vi "Wait.Gui.vi"() -> ()   [LabVIEW 2016]
uses:
  Wait.Gui.Action.ctl
  Global/ApplicationGlobal.vi
panel:
  in  "Open?":bool
  out "message":string
  out "_loop":i32(ring)=4
  out "status":string
  out "Slide":i32(slide) scale=-1.1..-1.0
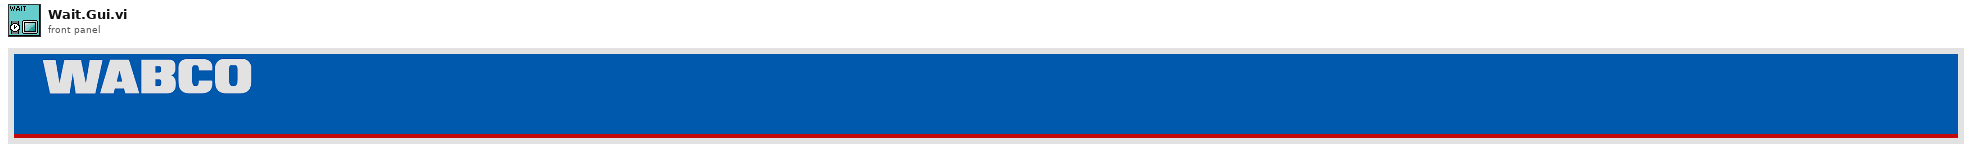
[diagram p1: front panel]
types:
  T1 = enum32{"Invalid", "Standard", "Closed", "Hidden", "Minimized", "Maximized"}
  T2 = enum32{"Invalid", "Default", "Floating", "Floating/Auto-Hide", "Modal"}
  T3 = cluster{"Msg":string, "Status":string, "ProgBarSize":i32, "Delay at open":u32}
  T4 = typedef "Wait.Gui.Action.ctl" = enum32{"idle", "constructor", "destructor", "--- WaitGui ---", "open FP", "close FP", "update msg", "update progbar"}
  T5 = typedef "LVPositionTypeDef.ctl" = cluster{"Left":i32, "Top":i32}
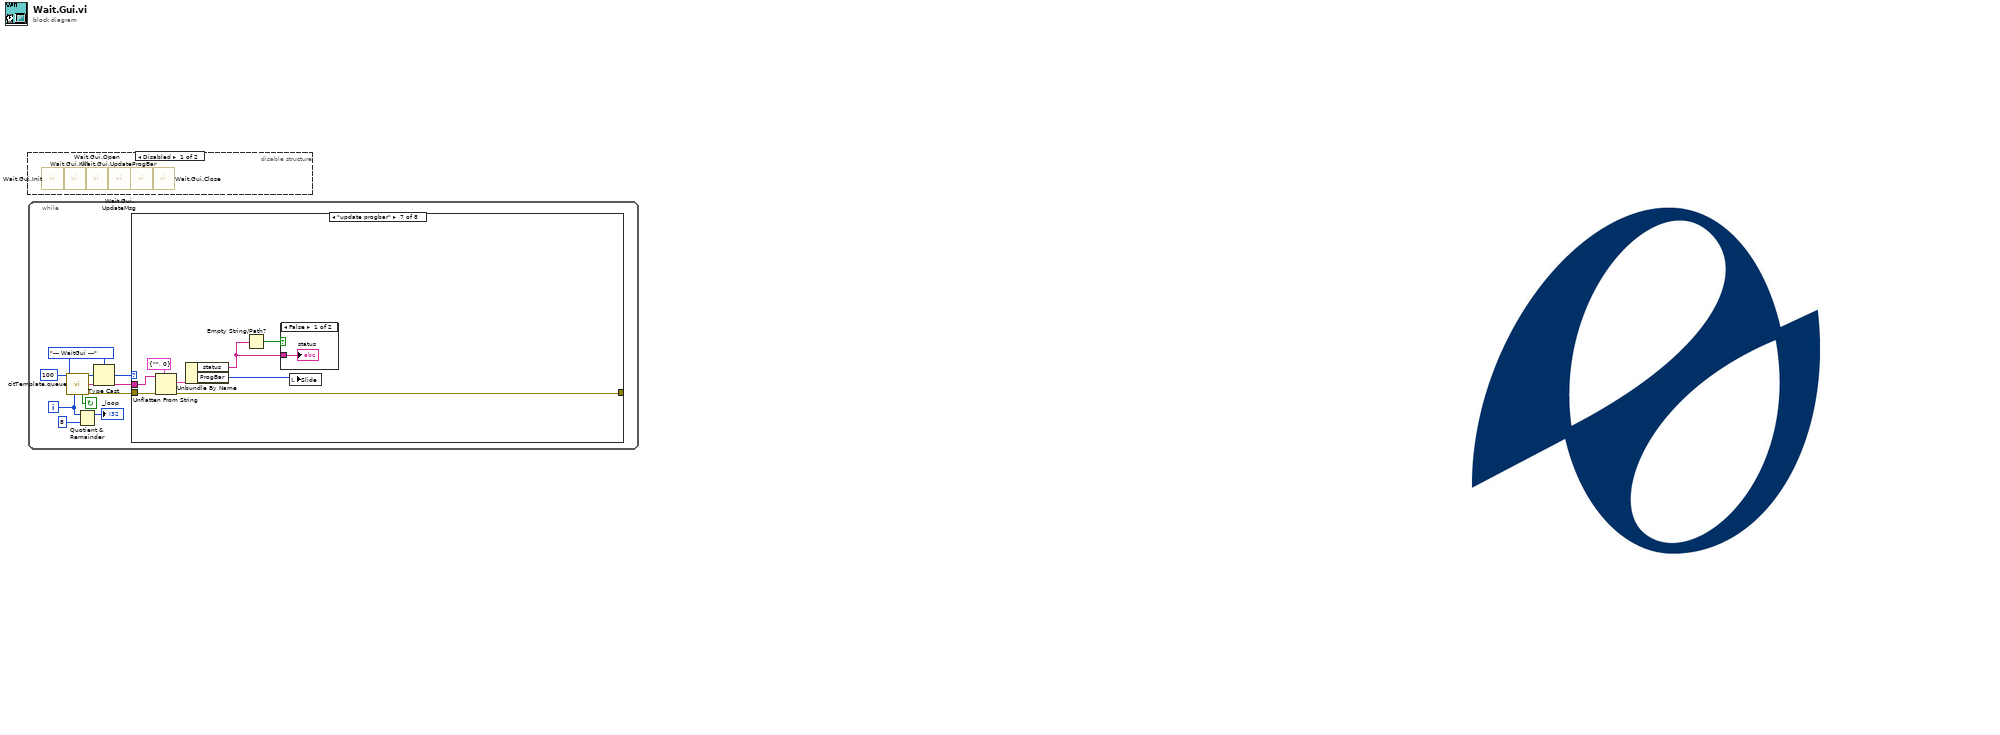
[diagram p0: block diagram]
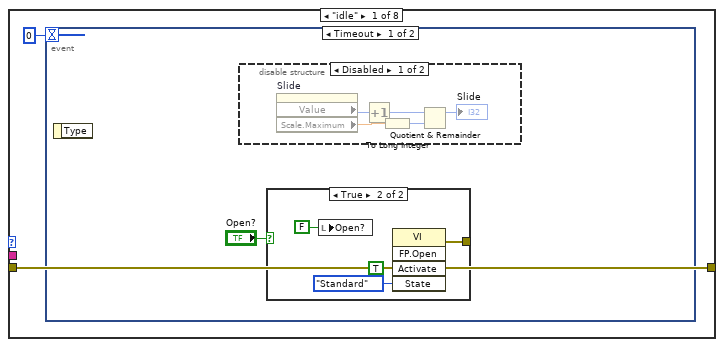
[diagram p3: hidden frame]
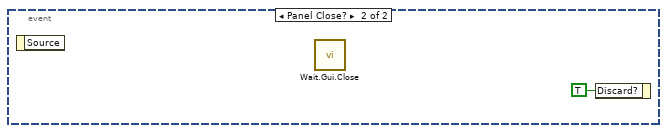
[diagram p6: hidden frame]
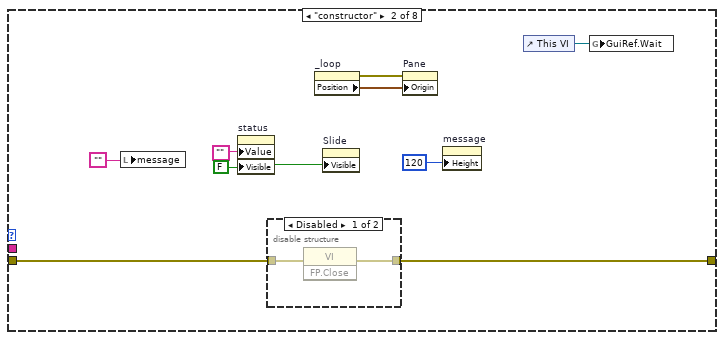
[diagram p7: hidden frame]
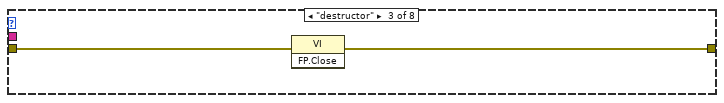
[diagram p9: hidden frame]
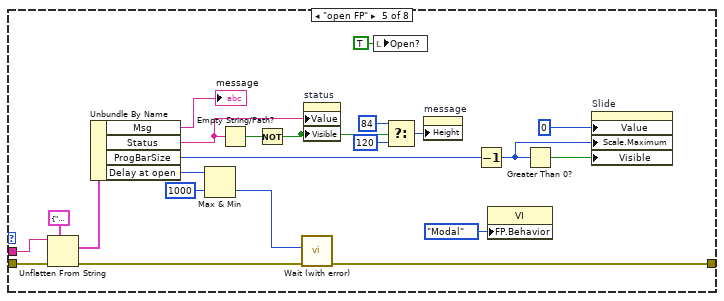
[diagram p11: hidden frame]
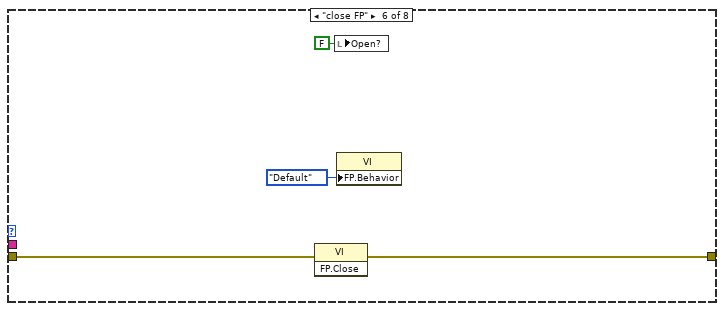
[diagram p12: hidden frame]
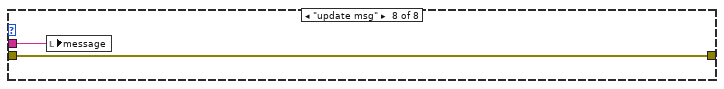
[diagram p14: hidden frame]
diagram:
  n1 = disable-structure shown="Disabled" {
    frame Disabled {
      n2 = call "Wait.Gui.Init.vi"() -> ()  [unwired: 11 in, 1 out]
      n3 = call "Wait.Gui.Kill.vi"() -> ()  [unwired: 11 in, 1 out]
      n4 = call "Wait.Gui.Open.vi"() -> ()  [unwired: 11 in, 1 out]
      n5 = call "Wait.Gui.UpdateMsg.vi"() -> ()  [unwired: 11 in, 1 out]
      n6 = call "Wait.Gui.UpdateProgBar.vi"() -> ()  [unwired: 11 in, 1 out]
      n7 = call "Wait.Gui.Close.vi"() -> ()  [unwired: 11 in, 1 out]
    }
    frame Enabled {
    }
  }
  n8 = while {
    i -> [w2]
    stop <- w4 continue-if-true
    w5 = Wait.Gui.Action."--- WaitGui ---" ("Action")
    n9 = call "citTemplate.queue.vi"("ms timeout (250 ms)"=100, "event enum"=w5, "iteration (-1)"=w2) -> ("event out"=w9:u32, "(flatten) data out"=w6:string, "continue"=w4:bool, "error out"=w7:errorcluster)  [unwired: 2 in, 7 out]
    n10 = Quotient & Remainder(x=w2, y=8) -> (x-y*floor(x/y)=→"_loop":i32)  [unwired: 1 out]
    n11 = Type Cast(type=w5, x=w9) -> (*(type *) &x=w8:T4)
    n12 = case shown="\"update progbar\"" w8 {
      tunnel: w7 -> [w11 w30 w37 w38 w60 w64 w72 w74]
      tunnel: w6 -> [_ _ _ _ w58 _ w71 w75]
      tunnel: [w11 w29 w36 w38 w42 w63 w70 w74] -> _
      frame "idle" {
        n13 = event shown="[0] Timeout" {
          selector: _ -> [_ _]
          dyn-events: _ -> [_ _]
          timeout: 0 -> [_ _]
          event Timeout {
            n14 = event-data() -> ()  [unwired: 1 in, 1 out]
            n15 = disable-structure shown="Disabled" {
              frame Disabled {
                n16 = property on="Slide" class="Slide (strict)"() -> ("Value"=w20:i32, "Scale.Maximum"=w21:dbl)  [unwired: 2 in, 2 out]
                n17 = Increment(x=w20) -> (x+1=w19:i32)
                n18 = To Long Integer(number=w21) -> (32bit integer=w22:i32)
                n19 = Quotient & Remainder(x=w19, y=w22) -> (x-y*floor(x/y)=→"Slide":i32)  [unwired: 1 out]
              }
              frame Enabled {
              }
            }
            n20 = case shown="True" "Open?" {
              tunnel: [_ w14] -> _
              frame False {
              }
              frame True {
                n21 = local write "Open?"(FALSE ("Open?")) -> ()
                n22 = invoke class="VI" method="FP.Open"("Activate"=TRUE ("Activate?"), "State"=T1."Standard") -> (error out=w14:errorcluster)  [unwired: 3 in, 4 out]
              }
            }
          }
          event Panel Close? {
            n23 = event-data() -> ()  [unwired: 1 in, 1 out]
            n24 = call "Wait.Gui.Close.vi"() -> ()  [unwired: 11 in, 1 out]
            n25 = event-data("Discard?"=TRUE) -> ()  [unwired: 1 in, 1 out]
          }
        }
      }
      frame "constructor" {
        w27 = FALSE ("Visible")
        n26 = local write "message"("") -> ()
        n27 = property on="status" class="Str"("Value"="", "Visible"=w27) -> ()  [unwired: 2 in, 2 out]
        n28 = disable-structure shown="Disabled" {
          disable-tunnel: w30 -> [w34 w35]
          disable-tunnel: [w33 w35] -> w29
          frame Disabled {
            n29 = invoke class="VI" method="FP.Close"(error in=w34) -> (error out=w33:errorcluster)  [unwired: 2 in, 2 out]
          }
          frame Enabled {
          }
        }
        n30 = property on="_loop" class="Ring (strict)"() -> (error out=w31:errorcluster, "Position"=w32:T5)  [unwired: 2 in, 1 out]
        n31 = property on="Slide" class="Slide (strict)"("Visible"=w27) -> ()  [unwired: 2 in, 2 out]
        n32 = property on="Pane" class="Pane"(error in=w31, "Origin"=w32) -> ()  [unwired: 1 in, 2 out]
        n33 = property on="message" class="Str"("Height"=u32 120 ("Size:Height")) -> ()  [unwired: 2 in, 2 out]
        n34 = control-ref of="This VI"() -> (w24:refnum<vi>)
        n35 = global write "ApplicationGlobal.vi" "GuiRef.Wait"(w24) -> ()
      }
      frame "destructor" {
        n36 = invoke class="VI" method="FP.Close"(error in=w37) -> (error out=w36:errorcluster)  [unwired: 2 in, 2 out]
      }
      frame "--- WaitGui ---" {
      }
      frame "open FP" {
        n37 = Unflatten From String(type=T3 {"Msg"="", "Status"="", "ProgBarSize"=0, "Delay at open"=0} ("output cluster"), binary string=w58, error in (no error)=w60) -> (value=w56:T3, error out=w59:errorcluster)  [unwired: 2 in, 1 out]
        n38 = Unbundle By Name(w56) -> ("Msg"=→"message":string, "Status"=w51:string, "ProgBarSize"=w55:i32, "Delay at open"=w45:u32)
        n39 = Max & Min(x=w45, y=u32 1000) -> (min(x,y)=w41:u32)  [unwired: 1 out]
        n40 = Empty String/Path?(string/path=w51) -> (empty?=w50:bool)
        n41 = Not(x=w50) -> (.not. x?=w46:bool)
        n42 = call "Wait (with error).vi"("error in (no error)"=w59, "milliseconds to wait"=w41) -> ("error out"=w42:errorcluster)  [unwired: 8 in, 1 out]
        n43 = property on="status" class="Str"("Value"=w51, "Visible"=w46) -> ()  [unwired: 2 in, 2 out]
        n44 = local write "Open?"(TRUE ("Wait")) -> ()
        n45 = Select(t=u32 84 ("Size:Height"), s=w46, f=u32 120 ("Size:Height")) -> (s? t:f=w49:u32)
        n46 = property on="message" class="Str"("Height"=w49) -> ()  [unwired: 2 in, 2 out]
        n47 = Decrement(x=w55) -> (x-1=w54:i32)
        n48 = property class="VI"("FP.Behavior"=T2."Modal" ("Front Panel Window:Behavior")) -> ()  [unwired: 2 in, 2 out]
        n49 = Greater Than 0?(x=w54) -> (x > 0?=w39:bool)
        n50 = property on="Slide" class="Slide (strict)"("Value"=0 ("Slide"), "Scale.Maximum"=w54, "Visible"=w39) -> ()  [unwired: 2 in, 2 out]
      }
      frame "close FP" {
        n51 = invoke class="VI" method="FP.Close"(error in=w64) -> (error out=w63:errorcluster)  [unwired: 2 in, 2 out]
        n52 = local write "Open?"(FALSE ("Wait")) -> ()
        n53 = property class="VI"("FP.Behavior"=T2."Default" ("Front Panel Window:Behavior")) -> ()  [unwired: 2 in, 2 out]
      }
      frame "update progbar" {
        n54 = Unflatten From String(type=cluster{"status":string, "ProgBar":i32} {"status"="", "ProgBar"=0} ("output cluster"), binary string=w71, error in (no error)=w72) -> (value=w68:cluster{"status":string, "ProgBar":i32}, error out=w70:errorcluster)  [unwired: 2 in, 1 out]
        n55 = Unbundle By Name(w68) -> ("status"=w65:string, "ProgBar"=w67:i32)
        n56 = Empty String/Path?(string/path=w65) -> (empty?=w66:bool)
        n57 = case shown="False" w66 {
          tunnel: w65 -> [w73 _]
          frame False {
            "status" <- w73
          }
          frame True {
          }
        }
        n58 = local write "Slide"(w67) -> ()
      }
      frame "update msg" {
        n59 = local write "message"(w75) -> ()
      }
    }
  }
